vi "Invalid Offset.vi"(7 "error source vi name":string, 8 "error in (no error)":errorcluster, 10 "offset":u64, 11 "Timing in":refnum<class "Timing.lvclass">) -> (0 "error out":errorcluster, 3 "Timing out":refnum<class "Timing.lvclass">)   [LabVIEW 2017, in "DSF Core.lvlib" / "Timing.lvclass"]
uses:
  Timing.lvclass
  Errors.ctl
  Timing.lvclass/Timing.ctl
  LabVIEW-Memory/Source/VIs/Source.Write.Scalar.Base10 (U64).vi
  LabVIEW-Memory/Source/Static Error Handling.lvlib
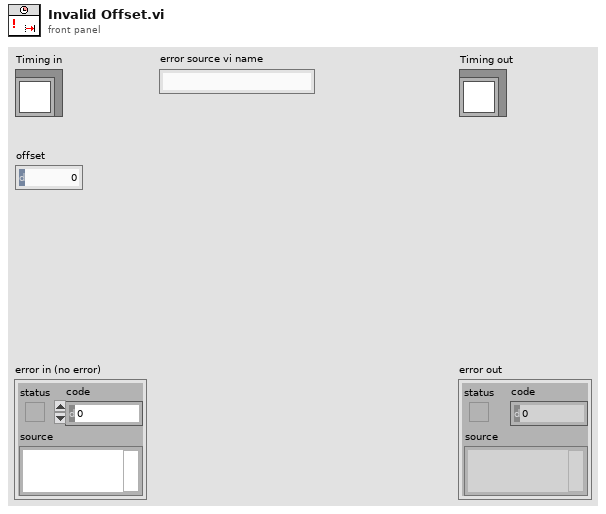
[diagram p1: front panel]
types:
  T1 = typedef "DSF Core.lvlib/Timing.lvclass/Errors.ctl" = enum16{"Invalid Offset", "Invalid Priority"}
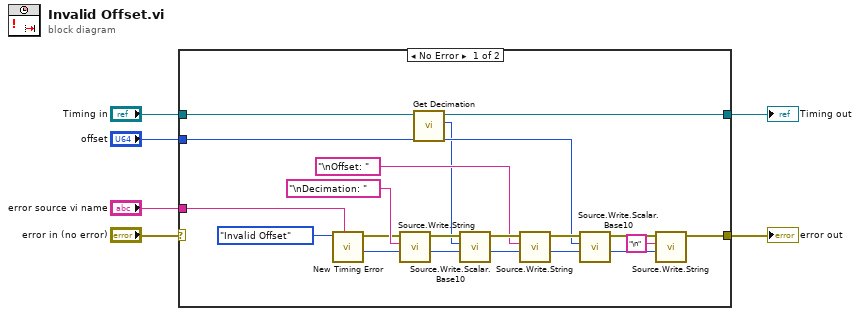
[diagram p0: block diagram]
diagram:
  n1 = case shown="No Error" "error in (no error)" {
    selector: "error in (no error)" -> [_ w27]
    tunnel: "Timing in" -> [w24 w28]
    tunnel: [w23 w28] -> w4
    tunnel: [w16 w27] -> w3
    tunnel: "error source vi name" -> [w25 _]
    tunnel: "offset" -> [w9 _]
    frame No Error {
      n2 = call "New Timing Error.vi"("error source vi name"=w25, "error"=Errors."Invalid Offset") -> ("new offset"=w15:i32, "error out"=w21:errorcluster)  [unwired: 8 in]
      n3 = call "Source.Write.String.vi"("offset"=w15, "string"="\nDecimation: ", "error in"=w21) -> ("new offset"=w14:i32, "error out"=w20:errorcluster)  [unwired: 7 in]
      n4 = call "Get Decimation.vi"("Timing in"=w24) -> ("Decimation"=w7:u64, "Timing out"=w23:refnum<class "Timing.lvclass">)  [unwired: 9 in]
      n5 = call-poly "Source.Write.Scalar.Base10.vi"("offset"=w14, "value"=w7, "error in"=w20) -> ("new offset"=w13:i32, "error out"=w19:errorcluster)  [unwired: 7 in]
      n6 = call "Source.Write.String.vi"("offset"=w13, "string"="\nOffset: ", "error in"=w19) -> ("new offset"=w12:i32, "error out"=w18:errorcluster)  [unwired: 7 in]
      n7 = call-poly "Source.Write.Scalar.Base10.vi"("offset"=w12, "value"=w9, "error in"=w18) -> ("new offset"=w11:i32, "error out"=w17:errorcluster)  [unwired: 7 in]
      n8 = call "Source.Write.String.vi"("offset"=w11, "string"="\n", "error in"=w17) -> ("error out"=w16:errorcluster)  [unwired: 7 in, 1 out]
    }
    frame Error {
    }
  }
  "error out" <- w3
  "Timing out" <- w4
